vi "Parameter Selection Dialog.vi"(7 "Param Size":enum16{"Scalar", "1d", "2d"}(ring), 8 "error in (no error)":errorcluster, 9 "NIVS.System Definition Root":refnum<k24>, 10 "NodePath":string) -> (0 "error out":errorcluster, 2 "Selected NodePath":string)   [LabVIEW 2011]
doc: "Use this template to create a dialog box with event handling."
uses:
  NationalInstruments.VeriStand.SystemStorageUI
  NationalInstruments.VeriStand.SystemStorage
  <vilib>/NI Veristand/UI Controls/Single Node Browser/NI_VS UI Single Node Browser.lvlib
panel:
  in  "Cancel":bool
  in  "Ok":bool
  in  "Parameter":refnum<k24>(container)
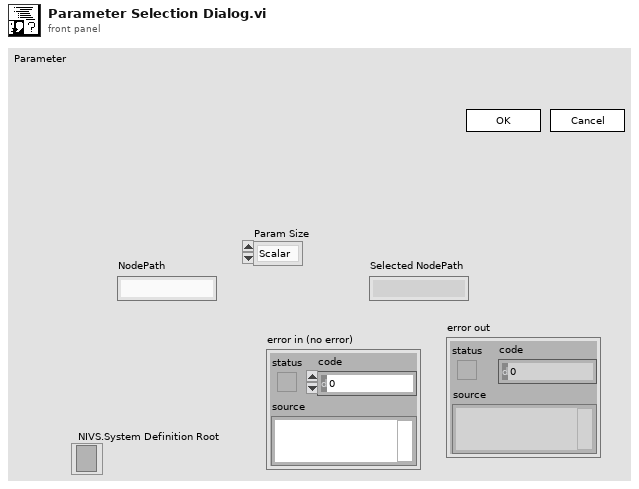
[diagram p1: front panel]
types:
  T1 = typedef "NI_VS UI Single Node Browser.lvlib/Callback Type.ctl" = cluster{"Net Callbacks":refnum<k27>[], "Event":refnum<user-event>}
  T2 = typedef "NI_VS UI Single Node Browser.lvlib/Node Ref.ctl" = refnum<k24>
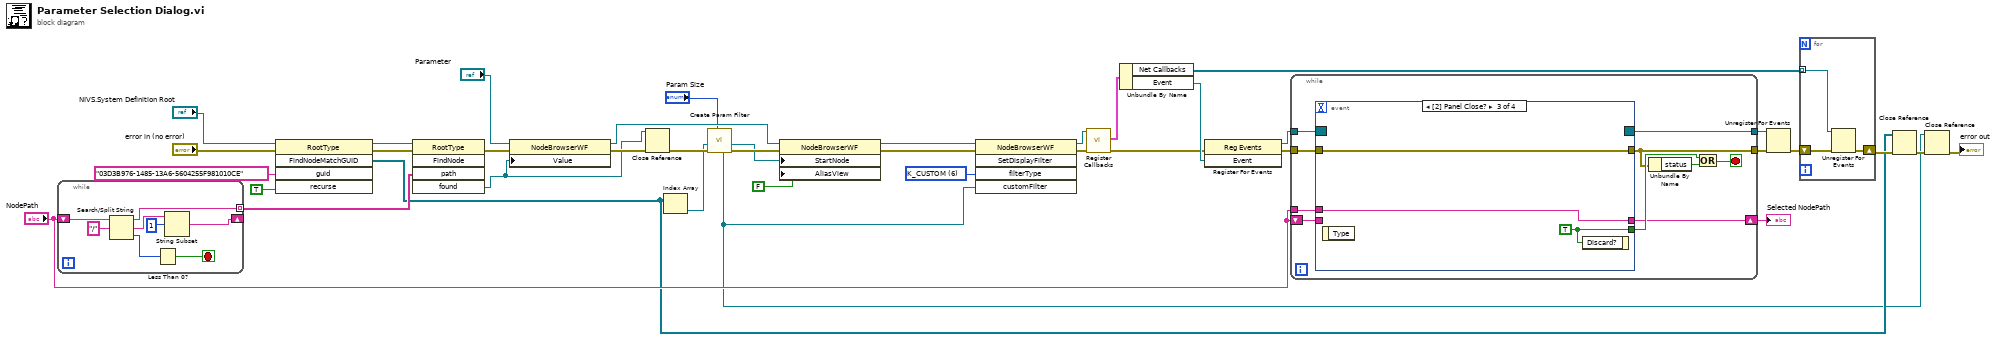
[diagram p0: block diagram]
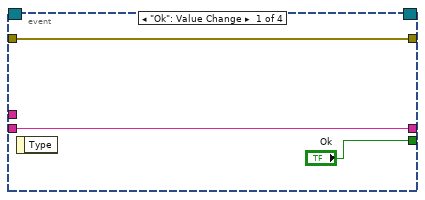
[diagram p2: hidden frame]
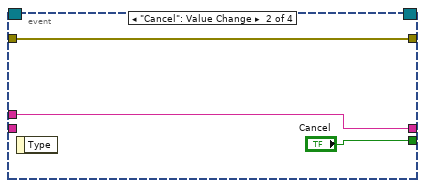
[diagram p3: hidden frame]
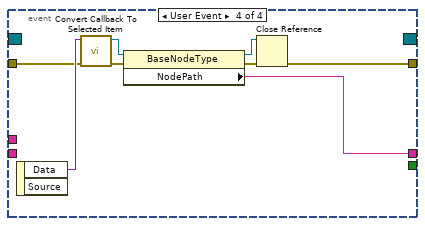
[diagram p4: hidden frame]
diagram:
  w15 = u8 6 items=["K_CHAN_R", "K_CHAN_W", "K_CHAN_RW", "K_CHAN_VOLT", "K_CHAN_FAULT", "K_ALL", "K_CUSTOM", "K_CHAN_R_VIS", "K_CHAN_W_VIS", "K_CHAN_RW_VIS", "K_CHAN_VOLT_VIS", "K_CHAN_FAULT_VIS"] ("filterType")
  n1 = while {
    tunnel: [w43] -> w23 mode=indexing
    shift-right: [w41] -> _
    shift-left: "NodePath" -> [w47]
    stop <- w44 stop-if-true
    n2 = Search/Split String(string=w47, search string/char (-)="/") -> (substring before match=w43:string, match + rest of string=w42:string, offset of match=w45:i32)  [unwired: 1 in]
    n3 = Less Than 0?(x=w45) -> (x < 0?=w44:bool)
    n4 = String Subset(string=w42, offset (0)=1) -> (substring=w41:string)  [unwired: 1 in]
  }
  n5 = invoke class="RootType" method="FindNodeMatchGUID"(reference="NIVS.System Definition Root", error in="error in (no error)", "guid"="03D3B976-1485-13A6-5604255F981010CE", "recurse"=TRUE) -> (reference out=w35:refnum<k24>, error out=w36:errorcluster, "FindNodeMatchGUID"=w11:refnum<k24>[])  [unwired: 1 in, 2 out]
  n6 = invoke class="RootType" method="FindNode"(reference=w35, error in=w36, "path"=w23) -> (error out=w32:errorcluster, "found"=w25:refnum<k24>)  [unwired: 2 in, 3 out]
  n7 = property class="NodeBrowserWF"(reference="Parameter", error in=w32, "Value"=w25) -> (reference out=w31:refnum<k24>, error out=w26:errorcluster)
  n8 = Close Reference(reference=w25, error in (no error)=w26) -> (error out=w10:errorcluster)
  n9 = Index Array(array=w11) -> (element=w4:refnum<k24>)  [unwired: 1 in]
  n10 = call "Create Param Filter.vi"("Param Size"="Param Size", "error in"=w10, "Model Section"=w4) -> ("error out"=w9:errorcluster, "Model Section dup"=w3:refnum<k24>, "Filter"=w2:refnum<k24>)  [unwired: 6 in]
  n11 = property class="NodeBrowserWF"(reference=w31, error in=w9, "StartNode"=w3, "AliasView"=FALSE) -> (reference out=w16:refnum<k24>, error out=w8:errorcluster)
  n12 = invoke class="NodeBrowserWF" method="SetDisplayFilter"(reference=w16, error in=w8, "filterType"=w15, "customFilter"=w2) -> (reference out=w17:refnum<k24>, error out=w18:errorcluster)  [unwired: 1 in, 3 out]
  n13 = call <vilib>:"Register Callbacks.vi"("error in (no error)"=w18, "Single Node Browser"=w17) -> ("error out"=w7:errorcluster, "Callbacks"=w34:T1)  [unwired: 7 in, 1 out]
  n14 = Unbundle By Name(w34) -> ("Net Callbacks"=w19:refnum<k27>[], "Event"=w29:refnum<user-event>)
  n15 = register-events(error in=w7, w29) -> (reference out=w39:refnum<event-registration>, error out=w27:errorcluster)  [unwired: 1 in]
  n16 = while {
    tunnel: [w55] -> w22
    tunnel: w27 -> [w56]
    tunnel: w39 -> [w52]
    shift-right: [w51] -> w28
    shift-left: "NodePath" -> [w50]
    tunnel: "NodePath" -> [w49]
    tunnel: [w48] -> w21
    stop <- w54 stop-if-true
    n17 = event shown="[2] Panel Close?" {
      selector: w52 -> [_ _ _ _]
      dyn-events: [_ _ _ _] -> w48
      timeout: _ -> [_ _ _ _]
      tunnel: ["Ok" "Cancel" w66 _] -> w57
      tunnel: [w60 w62 w65 w72] -> w55
      tunnel: w56 -> [w60 w62 w65 w73]
      tunnel: [w58 w61 w64 w67] -> w51
      tunnel: w50 -> [w58 _ _ _]
      tunnel: w49 -> [_ w61 w64 _]
      event "Ok": Value Change {
        n18 = event-data() -> ()  [unwired: 1 in, 1 out]
      }
      event "Cancel": Value Change {
        n19 = event-data() -> ()  [unwired: 1 in, 1 out]
      }
      event Panel Close? {
        w66 = TRUE ("Cancel")
        n20 = event-data() -> ()  [unwired: 1 in, 1 out]
        n21 = event-data("Discard?"=w66) -> ()  [unwired: 1 in, 1 out]
      }
      event User Event {
        n22 = event-data() -> ("Data"=w74:variant)  [unwired: 1 in, 1 out]
        n23 = call <vilib>:"Convert Callback To Selected Item.vi"("error in"=w73, "Data"=w74) -> ("error out"=w68:errorcluster, "Selected Item"=w71:T2)  [unwired: 8 in]
        n24 = property class="BaseNodeType"(reference=w71, error in=w68) -> (reference out=w70:T2, error out=w69:errorcluster, "NodePath"=w67:string)
        n25 = Close Reference(reference=w70, error in (no error)=w69) -> (error out=w72:errorcluster)
      }
    }
    n26 = Unbundle By Name(w55) -> ("status"=w53:bool)
    n27 = Or(x=w57, y=w53) -> (x .or. y?=w54:bool)
  }
  "Selected NodePath" <- w28
  n28 = Unregister For Events(event registration refnum=w21, error in=w22) -> (error out=w20:errorcluster)
  n29 = for {
    tunnel: w19 -> [w76] mode=indexing
    shift-right: [w75] -> w12
    shift-left: w20 -> [w77]
    n30 = Unregister For Events(event registration refnum=w76, error in=w77) -> (error out=w75:errorcluster)
  }
  n31 = Close Reference(reference=w11, error in (no error)=w12) -> (error out=w6:errorcluster)
  n32 = Close Reference(reference=w2, error in (no error)=w6) -> (error out=→"error out":errorcluster)
